vi "target4.vi"() -> ()   [LabVIEW 2023]
panel:
  in  "size":i32=100
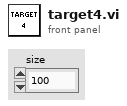
[diagram p1: front panel]
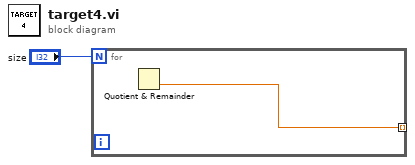
[diagram p0: block diagram]
diagram:
  n1 = for {
    N: "size" -> [_]
    tunnel: [w2] -> _ mode=indexing
    n2 = Quotient & Remainder() -> (floor(x/y)=w2:dbl)  [unwired: 2 in, 1 out]
  }
